vi "open_DAQmax_ports.vi"(8 "error in (no error)":errorcluster, 10 "UT/PASS/FAIL states":tag="Dev3/port1/line0:7", 11 "START/STOP buttons":tag="Dev3/port0/line0:7") -> (0 "error out":errorcluster, 2 "UT/PASS/FAIL states out":refnum<k21>, 3 "START/STOP buttons out":refnum<k21>)   [LabVIEW 2015]
uses:
  <vilib>/DAQmx/create/channels.llb/DAQmx Create Channel (DI-Digital Input).vi
  <vilib>/DAQmx/create/channels.llb/DAQmx Create Channel (DO-Digital Output).vi
panel:
  # "pot0=output"
  # "port1=input"
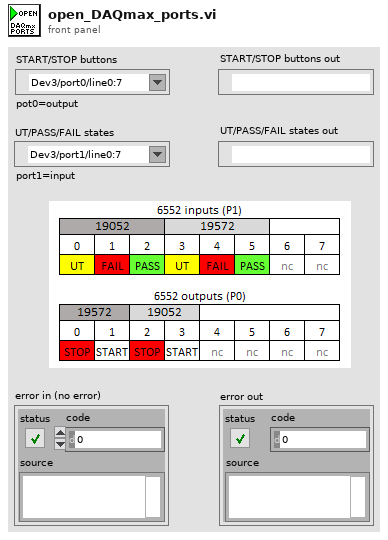
[diagram p1: front panel]
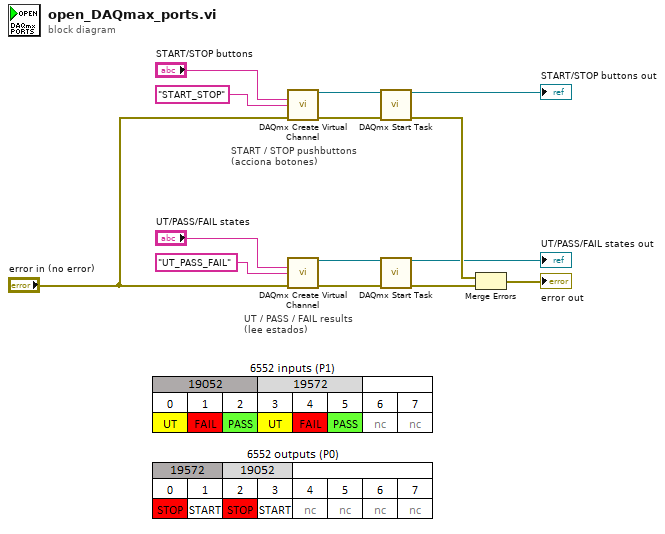
[diagram p0: block diagram]
diagram:
  # "UT / PASS / FAIL results\n(lee estados)"
  # "START / STOP pushbuttons\n(acciona botones)"
  n1 = call-poly <vilib>:"DAQmx Create Virtual Channel.vi"("lines"="START/STOP buttons", "name to assign"="START_STOP", "error in"="error in (no error)") -> ("task out"=w6:refnum<k21>, "error out"=w11:errorcluster)  [unwired: 11 in]
  n2 = call-poly <vilib>:"DAQmx Create Virtual Channel.vi"("lines"="UT/PASS/FAIL states", "name to assign"="UT_PASS_FAIL", "error in"="error in (no error)") -> ("task out"=w8:refnum<k21>, "error out"=w9:errorcluster)  [unwired: 11 in]
  n3 = call <vilib>:"DAQmx Start Task.vi"("task/channels in"=w6, "error in"=w11) -> ("task out"=→"START/STOP buttons out":refnum<k21>, "error out"=w12:errorcluster)  [unwired: 12 in]
  n4 = call <vilib>:"DAQmx Start Task.vi"("task/channels in"=w8, "error in"=w9) -> ("task out"=→"UT/PASS/FAIL states out":refnum<k21>, "error out"=w10:errorcluster)  [unwired: 12 in]
  n5 = Merge Errors(w12, w10) -> (→"error out":errorcluster)
